vi "FTP.GetLastFile.vi"(8 "error in (no error)":errorcluster, 10 "LogPath":path=path "C:/SOFTWARE/logs/scanner", 11 "FTP Session in":T1) -> (0 "error out":errorcluster, 2 "File name":path, 3 "FTP Session out":T1)   [LabVIEW 2016]
uses:
  <vilib>/FTP/ftp0.llb/FTP Session.ctl
  <vilib>/FTP/NI_FTP.lvlib
panel:
  out "Files":string[](array[string])
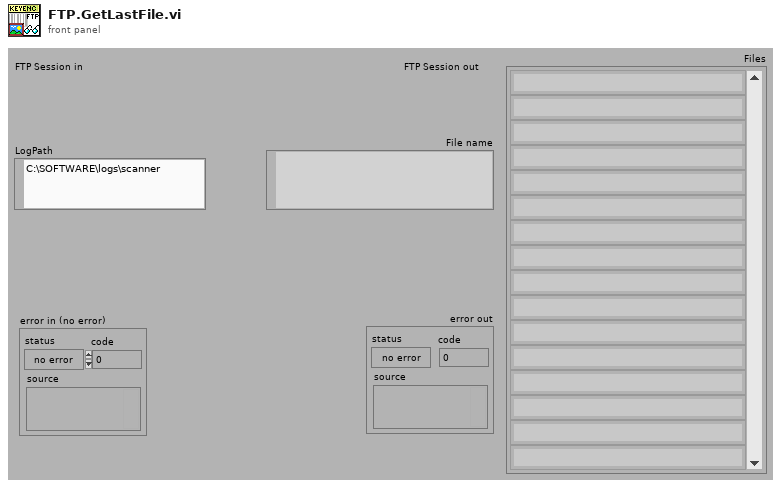
[diagram p1: front panel]
types:
  T1 = typedef "NI_FTP.lvlib/FTP Session.ctl" = refnum<k5>
  T2 = typedef "NI_FTP.lvlib/FTP File Info.ctl" = cluster{"type":enum16{"unknown", "file", "dir", "link"}, "permissions":string, "owner":string, "group":string, "size":i32, "date":string, "name":string, "link name":string}
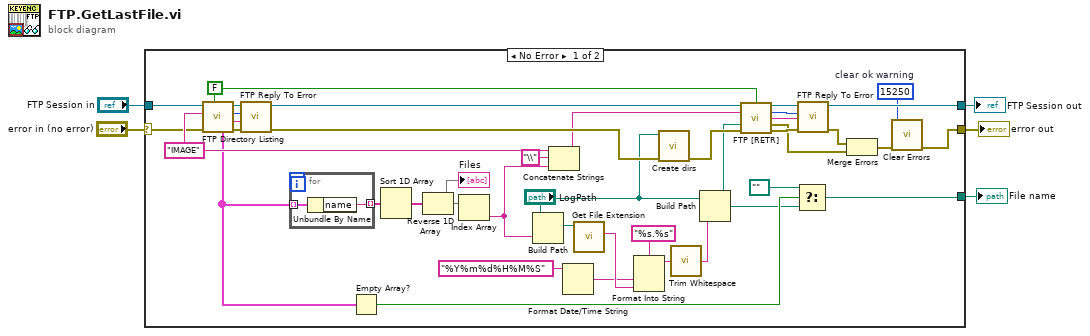
[diagram p0: block diagram]
diagram:
  n1 = case shown="No Error" "error in (no error)" {
    selector: "error in (no error)" -> [w14 w49]
    tunnel: [w7 w49] -> w5
    tunnel: [w17 _] -> w3
    tunnel: "FTP Session in" -> [w15 w48]
    tunnel: [w11 w48] -> w1
    frame No Error {
      w6 = 15250  # clear ok warning
      w22 = "IMAGE" ("directory path")
      w40 = FALSE ("active (T)")
      n2 = call <vilib>:"FTP Directory Listing.vi"("active (T)"=w40, "error in (no error)"=w14, "directory path"=w22, "ftp session"=w15) -> ("error out"=w44:errorcluster, "reply string"=w42:string, "reply code"=w43:i32, "ftp session out"=w45:T1, "dir list"=w20:T2[])  [unwired: 3 in]
      n3 = call <vilib>:"FTP Reply To Error.vi"("error in (no error)"=w44, "reply string in"=w42, "reply code in"=w43, "ftp session"=w45) -> ("error out"=w30:errorcluster, "ftp session out"=w41:T1)  [unwired: 2 out]
      n4 = for {
        tunnel: w20 -> [w47] mode=indexing
        tunnel: [w46] -> w25 mode=indexing
        n5 = Unbundle By Name(w47) -> ("name"=w46:string)
      }
      n6 = Empty Array?(array=w20) -> (empty?=w19:bool)
      n7 = Sort 1D Array(array=w25) -> (sorted array=w24:string[])
      n8 = Reverse 1D Array(array=w24) -> (reversed array=w8:string[])
      "Files" <- w8
      n9 = Index Array(array=w8) -> (element=w23:string)  [unwired: 1 in]
      n10 = Build Path(base path="LogPath", name or relative path=w23) -> (appended path=w35:path)
      n11 = Concatenate Strings(w22, "\\" ("string"), w23) -> (w26:string)
      n12 = Format Date/Time String(time format string (%c)="%Y%m%d%H%M%S") -> (date/time string=w12:string)  [unwired: 2 in]
      n13 = call <vilib>:"Get File Extension.vi"("file"=w35) -> ("lowercase file extension"=w27:string)  [unwired: 6 in, 4 out]
      n14 = Format Into String(format string="%s.%s", w12, w27) -> (resulting string=w34:string)  [unwired: 2 in, 1 out]
      n15 = call "Create dirs.vi"("error in (no error)"=w30, "deepest dir"="LogPath") -> ("error"=w29:errorcluster)  [unwired: 9 in]
      n16 = call <vilib>:"Trim Whitespace.vi"("string"=w34) -> ("trimmed string"=w32:string)  [unwired: 1 in]
      n17 = Build Path(base path="LogPath", name or relative path=w32) -> (appended path=w18:path)
      n18 = call <vilib>:"FTP [RETR].vi"("ftp session"=w41, "active (T)"=w40, "remote path"=w26, "local path (<NAP>)"=w18, "error in (no error)"=w29) -> ("ftp session out"=w39:T1, "reply code"=w37:i32, "reply string"=w36:string, "file error"=w33:errorcluster, "error out"=w38:errorcluster)  [unwired: 1 in, 5 out]
      n19 = Select(t=path "", s=w19, f=w18) -> (s? t:f=w17:path)
      n20 = call <vilib>:"FTP Reply To Error.vi"("error in (no error)"=w38, "reply string in"=w36, "reply code in"=w37, "ftp session"=w39) -> ("error out"=w10:errorcluster, "ftp session out"=w11:T1)  [unwired: 2 out]
      n21 = Merge Errors(w10, w33) -> (w9:errorcluster)
      n22 = call <vilib>:"Clear Errors.vi"("error in (no error)"=w9, "specific error code to clear (0: all)"=w6) -> ("error out"=w7:errorcluster)  [unwired: 4 in, 1 out]
    }
    frame Error {
    }
  }
  "error out" <- w5
  "File name" <- w3
  "FTP Session out" <- w1
